vi "Multiline String to Array (Preserve EOLs).vi"(1 "Input String":string) -> (0 "Array":string[](array[string]))   [LabVIEW 2013]
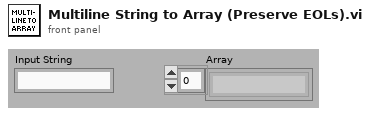
[diagram p1: front panel]
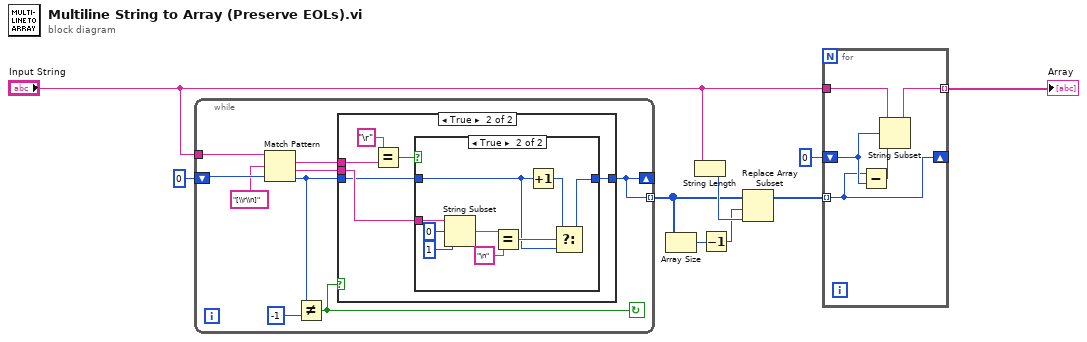
[diagram p0: block diagram]
diagram:
  n1 = while {
    tunnel: "Input String" -> [w18]
    shift-right: [w10] -> _
    shift-left: 0 ("offset past match") -> [w17]
    tunnel: [w10] -> w4 mode=indexing
    stop <- w11 continue-if-true
    n2 = Match Pattern(string=w18, regular expression="[\\r\\n]", offset (0)=w17) -> (match substring=w15:string, after substring=w14:string, offset past match=w12:i32)  [unwired: 1 out]
    n3 = Not Equal?(x=w12, y=-1) -> (x != y?=w11:bool)
    n4 = case shown="True" w11 {
      tunnel: w15 -> [_ w20]
      tunnel: w14 -> [_ w24]
      tunnel: w12 -> [w19 w22]
      tunnel: [w19 w21] -> w10
      frame False {
      }
      frame True {
        n5 = Equal?(x="\r" ("regular expression"), y=w20) -> (x = y?=w23:bool)
        n6 = case shown="True" w23 {
          tunnel: w24 -> [_ w35]
          tunnel: w22 -> [w26 w29]
          tunnel: [w26 w28] -> w21
          frame False {
          }
          frame True {
            n7 = String Subset(string=w35, offset (0)=0, length (rest)=1 ("length (rest)")) -> (substring=w32:string)
            n8 = Equal?(x=w32, y="\n" ("regular expression")) -> (x = y?=w30:bool)
            n9 = Increment(x=w29) -> (x+1=w27:i32)
            n10 = Select(t=w27, s=w30, f=w29) -> (s? t:f=w28:i32)
          }
        }
      }
    }
  }
  n11 = Array Size(array=w4) -> (size(s)=w5:i32)
  n12 = String Length(string="Input String") -> (length=w8:i32)
  n13 = Decrement(x=w5) -> (x-1=w6:i32)
  n14 = Replace Array Subset(array=w4, new element=w8, index=w6) -> (w2:i32[])
  n15 = for {
    tunnel: w2 -> [w36] mode=indexing
    tunnel: "Input String" -> [w40]
    shift-right: [w36] -> _
    shift-left: 0 ("offset past match") -> [w38]
    tunnel: [w37] -> w9 mode=indexing
    n16 = Subtract(x=w36, y=w38) -> (x-y=w39:i32)
    n17 = String Subset(string=w40, offset (0)=w38, length (rest)=w39) -> (substring=w37:string)
  }
  "Array" <- w9
